vi "MTMount_putSample_OSS4.vi"(8 "error in (no error)":errorcluster, 11 "OSS4_Ctl":T1) -> (0 "error out":errorcluster, 2 "function return":i32, 3 "OSS4_Ctl out":T1)   [LabVIEW 2018, in "SALLV_MTMount.lvlib"]
doc: "int MTMount_shm_putSample_OSS4LV(MTMount_OSS4LV *OSS4_Ctl );"
uses:
  SALLV_MTMount.lvlib
  DataTypes/OSS4.ctl
  SALLV_MTMount.so
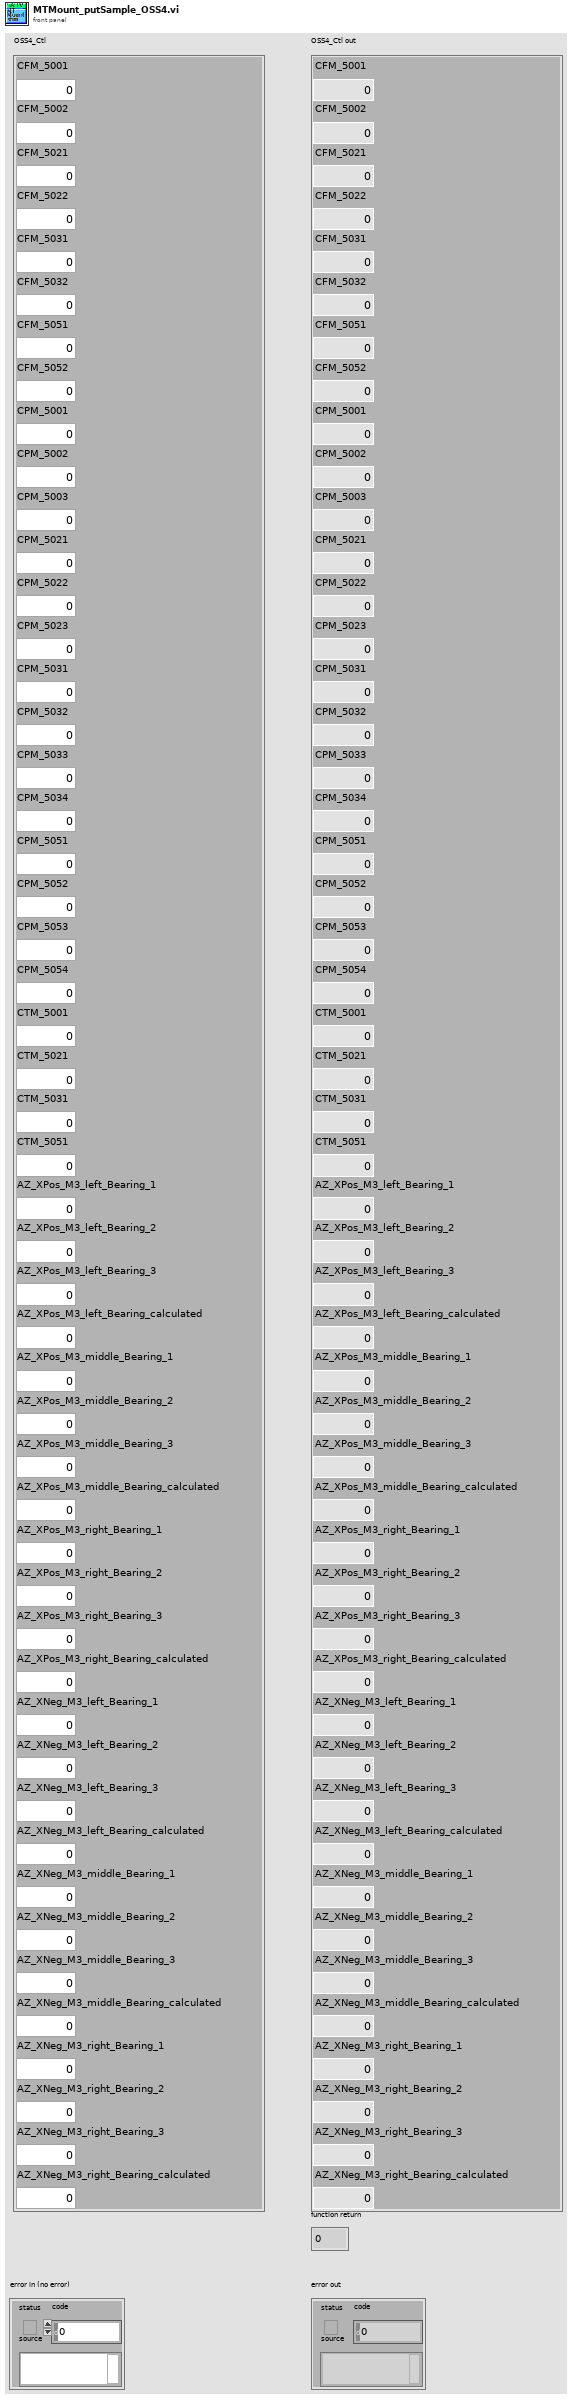
[diagram p1: front panel]
types:
  T1 = typedef "SALLV_MTMount.lvlib/OSS4.ctl" = cluster{"CFM_5001":dbl, "CFM_5002":dbl, "CFM_5021":dbl, "CFM_5022":dbl, "CFM_5031":dbl, "CFM_5032":dbl, "CFM_5051":dbl, "CFM_5052":dbl, "CPM_5001":dbl, "CPM_5002":dbl, "CPM_5003":dbl, "CPM_5021":dbl, "CPM_5022":dbl, "CPM_5023":dbl, "CPM_5031":dbl, "CPM_5032":dbl, "CPM_5033":dbl, "CPM_5034":dbl, "CPM_5051":dbl, "CPM_5052":dbl, "CPM_5053":dbl, "CPM_5054":dbl, "CTM_5001":dbl, "CTM_5021":dbl, "CTM_5031":dbl, "CTM_5051":dbl, "AZ_XPos_M3_left_Bearing_1":dbl, "AZ_XPos_M3_left_Bearing_2":dbl, "AZ_XPos_M3_left_Bearing_3":dbl, "AZ_XPos_M3_left_Bearing_calculated":dbl, "AZ_XPos_M3_middle_Bearing_1":dbl, "AZ_XPos_M3_middle_Bearing_2":dbl, "AZ_XPos_M3_middle_Bearing_3":dbl, "AZ_XPos_M3_middle_Bearing_calculated":dbl, "AZ_XPos_M3_right_Bearing_1":dbl, "AZ_XPos_M3_right_Bearing_2":dbl, "AZ_XPos_M3_right_Bearing_3":dbl, "AZ_XPos_M3_right_Bearing_calculated":dbl, "AZ_XNeg_M3_left_Bearing_1":dbl, "AZ_XNeg_M3_left_Bearing_2":dbl, "AZ_XNeg_M3_left_Bearing_3":dbl, "AZ_XNeg_M3_left_Bearing_calculated":dbl, "AZ_XNeg_M3_middle_Bearing_1":dbl, "AZ_XNeg_M3_middle_Bearing_2":dbl, "AZ_XNeg_M3_middle_Bearing_3":dbl, "AZ_XNeg_M3_middle_Bearing_calculated":dbl, "AZ_XNeg_M3_right_Bearing_1":dbl, "AZ_XNeg_M3_right_Bearing_2":dbl, "AZ_XNeg_M3_right_Bearing_3":dbl, "AZ_XNeg_M3_right_Bearing_calculated":dbl}
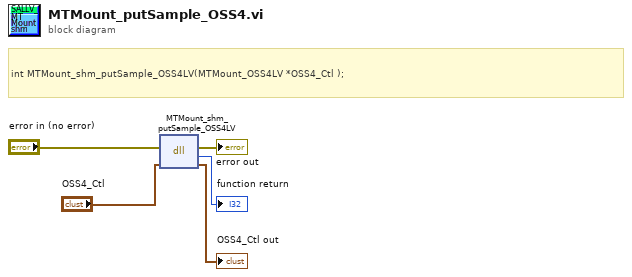
[diagram p0: block diagram]
diagram:
  # "int MTMount_shm_putSample_OSS4LV(MTMount_OSS4LV *OSS4_Ctl );"
  n1 = dll-call lib="home/ttsai/Document/salApiMTMount/SALLV_MTMount/SALLV_MTMount.*" fn="MTMount_shm_putSample_OSS4LV"(error in="error in (no error)", "OSS4_Ctl"="OSS4_Ctl") -> (error out=→"error out":errorcluster, →"function return":i32, "OSS4_Ctl"=→"OSS4_Ctl out":T1)  [unwired: 2 in, 1 out]
